vi "Main.vi"(8 "error in (no error)":errorcluster, 11 "STDF File Parser in":refnum<class "STDF File Parser.lvclass">) -> (0 "error out":errorcluster, 3 "STDF File Parser out":refnum<class "STDF File Parser.lvclass">)   [LabVIEW 2018, in "STDF File Parser.lvclass"]
uses:
  STDF File Parser.lvclass
  STDF File Parser.lvclass/STDF File Parser.ctl
  TestDataMgr/TestDataMgr.lvclass
  <userlib>/STDF/PTR/PTR.lvclass
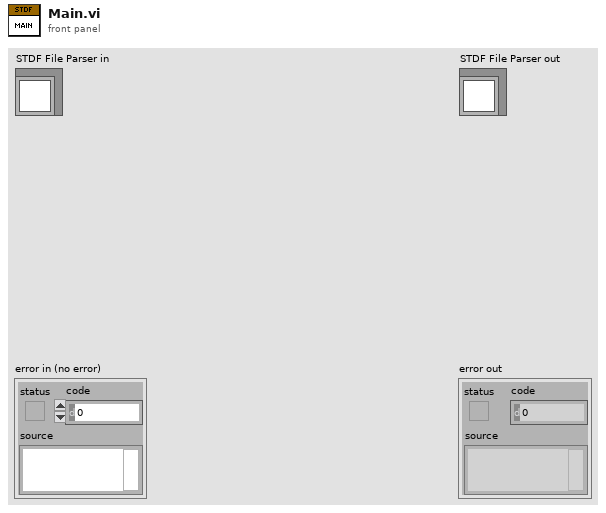
[diagram p1: front panel]
types:
  T1 = typedef "TestDataMgr.lvclass/Session Handle.ctl" = refnum<data-value>
  T2 = typedef "TestDataMgr.lvclass/Test Data All.ctl" = cluster{"Test Name":string, "Test Limits":T3, "Raw Data Per Tester":T4[]}
  T3 = typedef "TestDataMgr.lvclass/Test Limits.ctl" = cluster{"High":dbl, "Low":dbl}
  T4 = typedef "TestDataMgr.lvclass/Test Raw Data.ctl" = cluster{"Data":dbl[][], "Tester#":u8}
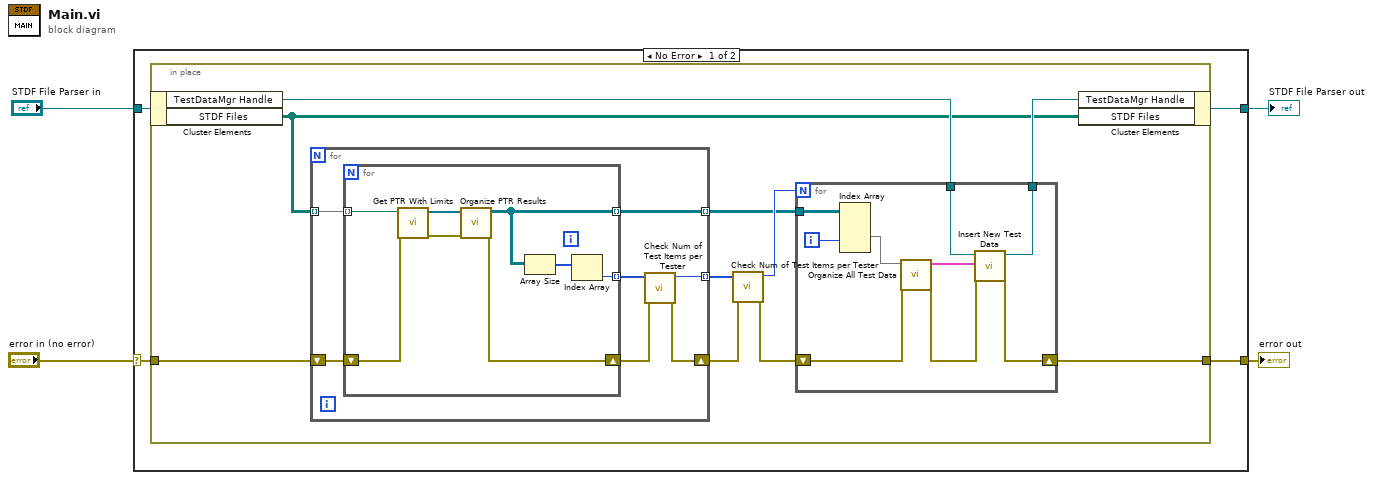
[diagram p0: block diagram]
diagram:
  n1 = case shown="No Error" "error in (no error)" {
    selector: "error in (no error)" -> [w8 w44]
    tunnel: [w5 w44] -> w3
    tunnel: [w6 w43] -> w1
    tunnel: "STDF File Parser in" -> [w7 w43]
    frame No Error {
      n2 = in-place {
        in-place-border: w8 -> [w18]
        in-place-border: [w15] -> w5
        n3 = in-place-cluster #1(w7) -> ("TestDataMgr Handle"=w17:T1, "STDF Files"=w14:path[][])
        n4 = for {
          shift-right: [w21] -> w12
          shift-left: w18 -> [w25]
          tunnel: w14 -> [w24] mode=indexing
          tunnel: [w20] -> w9 mode=indexing
          tunnel: [w19] -> w13 mode=indexing
          n5 = for {
            shift-right: [w30] -> w22
            shift-left: w25 -> [w33]
            tunnel: [w28] -> w23 mode=indexing
            tunnel: [w27] -> w20 mode=indexing
            tunnel: w24 -> [w26] mode=indexing
            n6 = call "Get PTR With Limits.vi"("error in"=w33, "Path to STDF file"=w26) -> ("error out"=w31:errorcluster, "PTRs W/Limits"=w32:refnum<class "PTR.lvclass">[])  [unwired: 8 in]
            n7 = call "Organize PTR Results.vi"("error in (no error)"=w31, "PTRs W/Limits"=w32) -> ("error out"=w30:errorcluster, "Sorted PTR"=w27:refnum<class "PTR.lvclass">[][])  [unwired: 8 in]
            n8 = Array Size(array=w27) -> (size(s)=w29:i32[])
            n9 = Index Array(array=w29) -> (element=w28:i32)  [unwired: 1 in]
          }
          n10 = call "Check Num of Test Items per Tester.vi"("Error in"=w22, "# of Test Item"=w23) -> ("Error out"=w21:errorcluster, "Num of Test Item"=w19:i32)  [unwired: 8 in]
        }
        n11 = call "Check Num of Test Items per Tester.vi"("Error in"=w12, "# of Test Item"=w13) -> ("Error out"=w10:errorcluster, "Num of Test Item"=w11:i32)  [unwired: 8 in]
        n12 = for {
          N: w11 -> [_]
          shift-right: [w38] -> w15
          shift-left: w10 -> [w40]
          tunnel: w17 -> [w42]
          tunnel: [w37] -> w16
          tunnel: w9 -> [w36]
          i -> [w35]
          n13 = Index Array(array=w36, index (dim 2)=w35) -> (element=w34:refnum<class "PTR.lvclass">[][][])  [unwired: 3 in]
          n14 = call "Organize All Test Data.vi"("error in (no error)"=w40, "Test Item PTR From All STDF"=w34) -> ("error out"=w39:errorcluster, "Test Data Out"=w41:T2)  [unwired: 8 in]
          n15 = call "Insert New Test Data.vi"("error in (no error)"=w39, "Test Data"=w41, "Session Handle in"=w42) -> ("error out"=w38:errorcluster, "Session Handle out"=w37:T1)  [unwired: 7 in]
        }
        n16 = in-place-cluster #1("TestDataMgr Handle"=w16, "STDF Files"=w14) -> (w6:refnum<class "STDF File Parser.lvclass">)
      }
    }
    frame Error {
    }
  }
  "error out" <- w3
  "STDF File Parser out" <- w1
